vi "Temperature Multiplot.vi"() -> ()   [LabVIEW 2014]
doc: "This VI is the solution to an exercise in the LabVIEW Core I course.\n\nIt is used to demonstrate While loops and waveform charts. This VI takes a temperature reading from the temperature sensor on the DAQ signal accessory once every 500 ms and plots the data in a strip chart."
panel:
  out "Temperature History":cluster{"Temperature":dbl, "Temperature":dbl}(graph)
  in  "Power":bool=TRUE
  # "ON\n\n\n\n\nOFF"
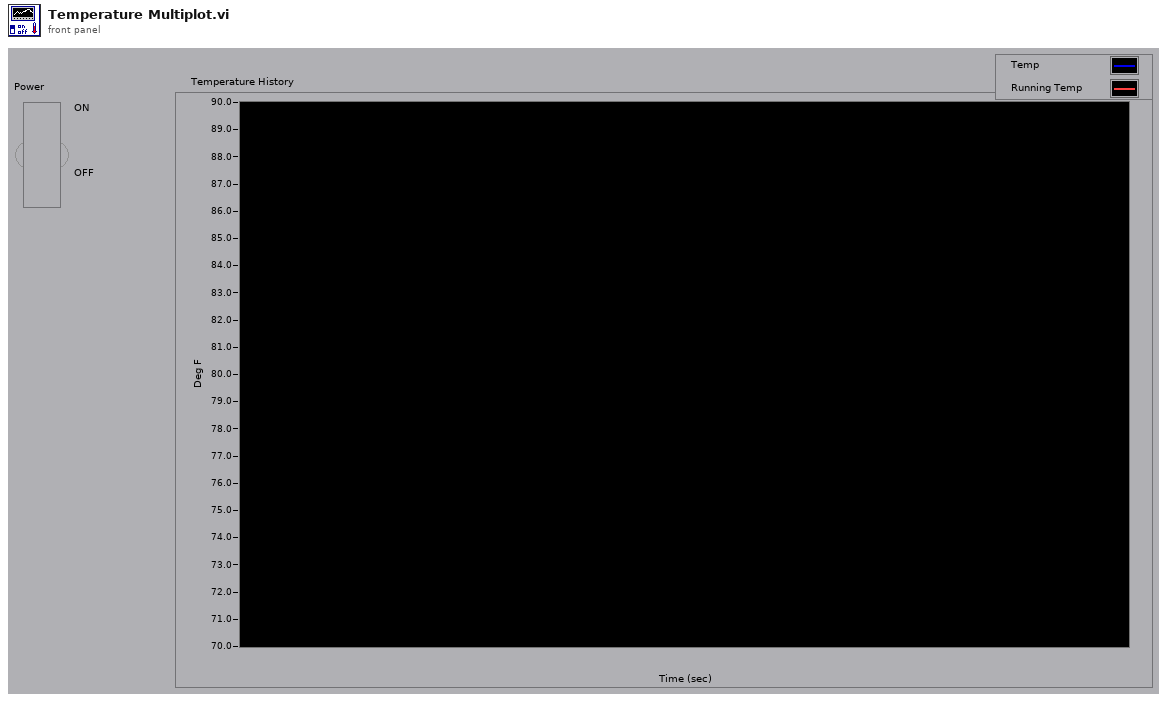
[diagram p1: front panel]
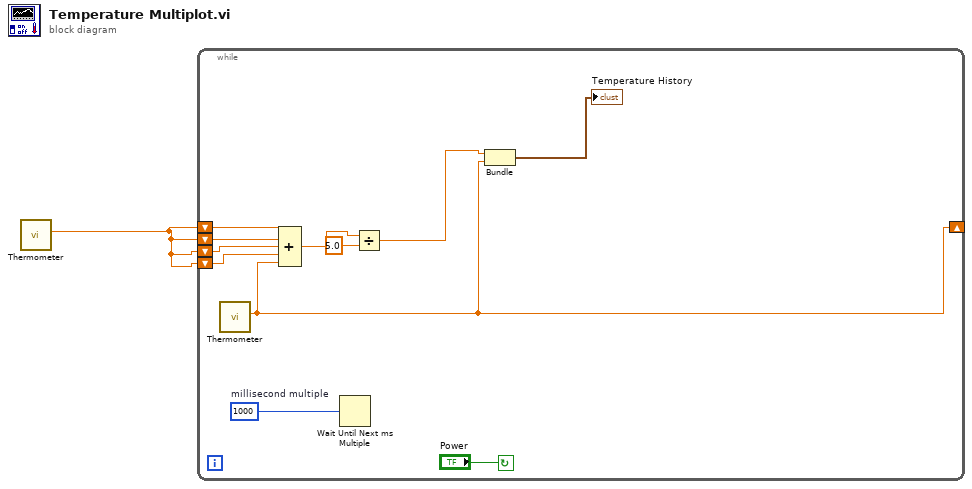
[diagram p0: block diagram]
diagram:
  n1 = call "Thermometer.vi"() -> ("Temperature"=w1:dbl)  [unwired: 10 in, 1 out]
  n2 = while {
    shift-right: [w2] -> _
    shift-left: w1 -> [w10]
    shift-left: w1 -> [w9]
    shift-left: w1 -> [w8]
    shift-left: w1 -> [w7]
    stop <- "Power" continue-if-true
    w11 = u32 1000  # millisecond multiple
    n3 = call "Thermometer.vi"() -> ("Temperature"=w2:dbl)  [unwired: 10 in, 1 out]
    n4 = Compound Arithmetic op=ADD(w10, w9, w8, w7, w2) -> (w5:dbl)
    n5 = Wait Until Next ms Multiple(millisecond multiple=w11) -> ()  [unwired: 1 out]
    n6 = Divide(x=w5, y=5.0) -> (x/y=w4:dbl)
    n7 = Bundle(w4, "Temperature"=w2) -> (→"Temperature History":cluster{dbl, "Temperature":dbl})  [unwired: 1 in]
  }
